vi "Untitled 1.vi"() -> ()   [LabVIEW 2019]
uses:
  <vilib>/Analysis/coordinate.llb/2D Cartesian Coordinate Rotation (Array).vi
  <vilib>/Analysis/NI_AALPro.lvlib
panel:
  out "Y Out":dbl[](array[numeric])
  out "X Out":dbl[](array[numeric])
  out "Y-CY":dbl
  out "X-CX":dbl
  out "y 2":dbl
  out "x 2":dbl
  out "Numeric":dbl
  out "theta Constant":dbl
  out "r":dbl
  out "y":dbl
  out "x":dbl
  out "CX":dbl
  out "CY":dbl
  out "R":dbl
  out "X":dbl
  out "Y":dbl
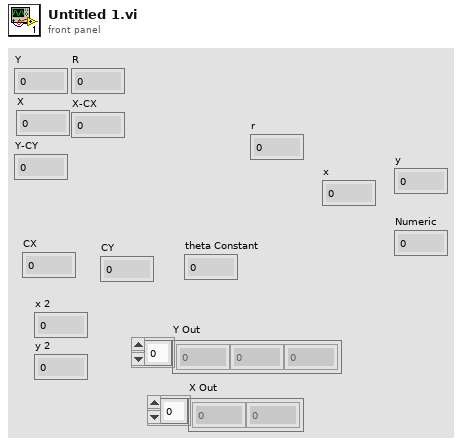
[diagram p1: front panel]
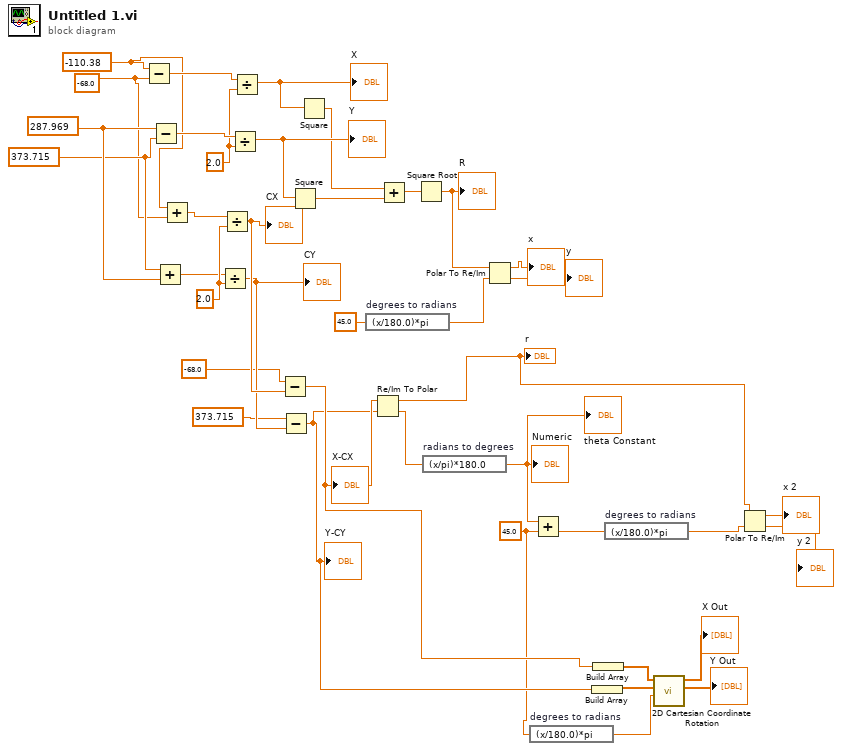
[diagram p0: block diagram]
diagram:
  w3 = 45.0 ("y")
  w31 = 2.0 ("y")
  w37 = 2.0 ("y")
  w20 = 373.715
  w29 = 287.969
  w22 = -110.38
  w19 = -68.0
  n1 = Subtract(x=w22, y=w19) -> (x-y=w39:dbl)
  n2 = Subtract(x=w29, y=w20) -> (x-y=w38:dbl)
  n3 = Add(x=w20, y=w29) -> (x+y=w28:dbl)
  n4 = Add(x=w22, y=w19) -> (x+y=w30:dbl)
  n5 = Divide(x=w28, y=w31) -> (x/y=w18:dbl)
  "CY" <- w18
  n6 = Divide(x=w30, y=w31) -> (x/y=w21:dbl)
  "CX" <- w21
  n7 = Divide(x=w38, y=w37) -> (x/y=w35:dbl)
  "Y" <- w35
  n8 = Divide(x=w39, y=w37) -> (x/y=w36:dbl)
  "X" <- w36
  n9 = Subtract(x=-68.0, y=w21) -> (x-y=w8:dbl)
  "X-CX" <- w8
  n10 = Subtract(x=373.715, y=w18) -> (x-y=w5:dbl)
  "Y-CY" <- w5
  n11 = Square(x=w35) -> (x^2=w33:dbl)
  n12 = Square(x=w36) -> (x^2=w34:dbl)
  n13 = expression code="(x/180.0)*pi" "degrees to radians"(45.0) -> (w26:dbl)
  n14 = Re/Im To Polar(2:w5, 3:w8) -> (0:w15:dbl, 1:w13:dbl)
  "r" <- w13
  n15 = Add(x=w34, y=w33) -> (x+y=w32:dbl)
  n16 = Square Root(x=w32) -> (sqrt(x)=w27:dbl)
  "R" <- w27
  n17 = expression code="(x/pi)*180.0" "radians to degrees"(w15) -> (w9:dbl)
  "theta Constant" <- w9
  "Numeric" <- w9
  n18 = Polar To Re/Im(2:w26, 3:w27) -> (0:→"y":dbl, 1:→"x":dbl)
  n19 = expression code="(x/180.0)*pi" "degrees to radians"(w3) -> (w4:dbl)
  n20 = Add(x=w9, y=w3) -> (x+y=w14:dbl)
  n21 = Build Array(w5) -> (w6:dbl[])
  n22 = Build Array(w8) -> (w7:dbl[])
  n23 = expression code="(x/180.0)*pi" "degrees to radians"(w14) -> (w12:dbl)
  n24 = call-poly <vilib>:"2D Cartesian Coordinate Rotation.vi"("theta"=w4, "Y"=w6, "X"=w7) -> ("Y Out"=→"Y Out":dbl[], "X Out"=→"X Out":dbl[])  [unwired: 6 in, 1 out]
  n25 = Polar To Re/Im(2:w12, 3:w13) -> (0:→"y 2":dbl, 1:→"x 2":dbl)
